vi "Configure Modulation (Binary-Phase-Shift Keying).vi"(0 "VISA resource name":refnum<visa-resource-name>, 1 "BPSK Source (0: Internal)":i32(ring) items=["Internal", "External"], 5 "Channel (1: 1)":i32(ring)=1 items=["1"=1, "2"=2], 7 "Enable BPSK Module(T: Enable)":bool=TRUE, 11 "error in (no error)":errorcluster, 12 "Modulation Phase Shift (180 Degree)":dbl=180.0, 13 "Modulation Rate (10 Hz)":dbl=10.0) -> (4 "VISA resource name out":refnum<visa-resource-name>, 15 "error out":errorcluster)   [LabVIEW 2019, in "Agilent 3352X Series.lvlib"]
doc: "Allows and configures Binary Phase Shift Keying(BPSK) modulation. Binary Phase Shift Keying (BPSK) is a digital modulation format. In BPSK, the carrier waveform is phase shifted between two phase settings using an on/off keying.\n\n<b>Note</b>:\n(1) When enabling this mode, all other modes will be turned off.\n(2) You can select a sine, square, ramp, or arbitrary waveform for the carrier (pulse, noise, PRBS, and DC are not allowed). \n(3) The carrier waveform parameters are set by the Configure Standard Waveform VI"
uses:
  <instrlib>/Agilent 3352X Series/Agilent 3352X Series.lvlib
panel:
  # "Internal BPSK Modulation Settings"
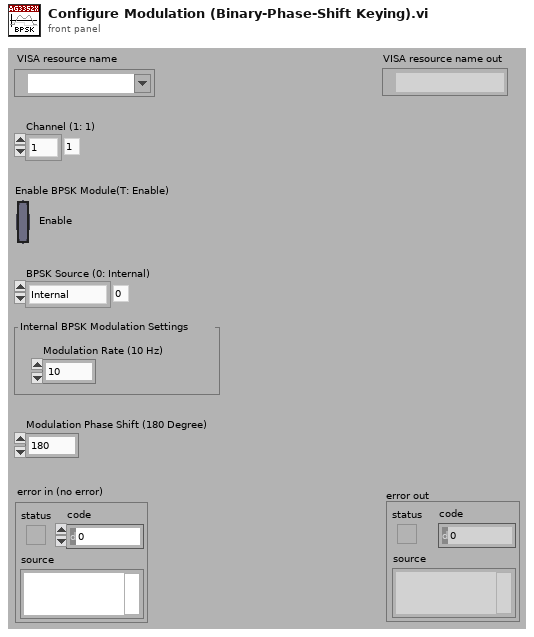
[diagram p1: front panel]
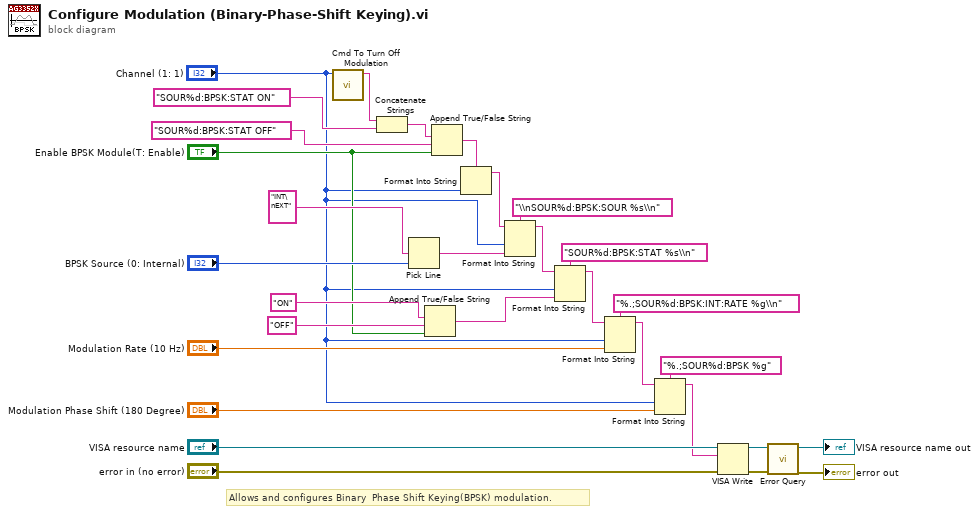
[diagram p0: block diagram]
diagram:
  # "Allows and configures Binary  Phase Shift Keying(BPSK) modulation."
  n1 = call <instrlib>:"Cmd To Turn Off Modulation.vi"("Channel (1: 1)"="Channel (1: 1)") -> ("Cmd String"=w5:string)  [unwired: 10 out]
  n2 = Concatenate Strings(w5, "SOUR%d:BPSK:STAT ON") -> (w8:string)
  n3 = Pick Line(multi-line string="INT\nEXT", line index="BPSK Source (0: Internal)") -> (output string=w27:string)  [unwired: 1 out]
  n4 = Append True/False String(1:"Enable BPSK Module(T: Enable)", 2:"OFF", 3:"ON") -> (0:w22:string)  [unwired: 1 out]
  n5 = Append True/False String(1:"Enable BPSK Module(T: Enable)", 2:"SOUR%d:BPSK:STAT OFF", 3:w8) -> (0:w7:string)  [unwired: 1 out]
  n6 = Format Into String(format string=w7, "Channel (1: 1)") -> (resulting string=w2:string)  [unwired: 2 in, 1 out]
  n7 = Format Into String(format string="\\nSOUR%d:BPSK:SOUR %s\\n", initial string=w2, "Channel (1: 1)", w27) -> (resulting string=w24:string)  [unwired: 1 in, 1 out]
  n8 = Format Into String(format string="SOUR%d:BPSK:STAT %s\\n", initial string=w24, "Channel (1: 1)", w22) -> (resulting string=w21:string)  [unwired: 1 in, 1 out]
  n9 = Format Into String(format string="%.;SOUR%d:BPSK:INT:RATE %g\\n", initial string=w21, "Channel (1: 1)", "Modulation Rate (10 Hz)") -> (resulting string=w18:string)  [unwired: 1 in, 1 out]
  n10 = Format Into String(format string="%.;SOUR%d:BPSK %g", initial string=w18, "Channel (1: 1)", "Modulation Phase Shift (180 Degree)") -> (resulting string=w9:string)  [unwired: 1 in, 1 out]
  n11 = VISA Write(VISA resource name="VISA resource name", write buffer=w9, error in (no error)="error in (no error)") -> (VISA resource name out=w13:refnum<visa-resource-name>, error out=w12:errorcluster)  [unwired: 1 out]
  n12 = call <instrlib>:"Error Query.vi"("error in (no error)"=w12, "VISA resource name"=w13) -> ("error out"=→"error out":errorcluster, "VISA resource name out"=→"VISA resource name out":refnum<visa-resource-name>)  [unwired: 8 out]
